vi "UART_SimpleExample.vi"() -> ()   [LabVIEW 2024, in "UART.lvlib"]
doc: "Simple example that shows how to send a command to the DUT and receive the response.\nThe DUT is powered up using a channel from the NI 657x board.\nThe command is sent in the form of Byte Array to be more generic as possible.\nThe response is also received an the form of Byte Array to be more generic as possible"
uses:
  UART.lvlib
panel:
  in  "Input Bytes":u8[](array[numeric])=[1, 3, 12, 0] format="%x"
  out "pass":bool[](array[boolean])=[TRUE]
  out "Reply Bytes":u8[](array[numeric])=[4, 14, 4, 1, 3, 12, 0] format="%x"
  out "error out":errorcluster
  in  "Pattern Label":string="Uart_Main"
  in  "Reply Bytes":i32=7
  in  "EOL Char (Hex)":u8 format="%x"
  in  "Source Buffer":i32=100
  in  "Pin Capture":string="UART_TX_07"
  in  "Pin Source":string="UART_RX_06"
  in  "levels file paths":path[](array[path])=[path "C:/Users/8880_AN/Documents/Customers/STM/657x_UART/DigitalPattern/Levels/LevelsDefault.digilevels"]
  in  "patterns file paths":path[](array[path])=[path "C:/Users/8880_AN/Documents/Customers/STM/657x_UART/DigitalPattern/Pattern/UART_Main.digipat", path "C:/Users/8880_AN/Documents/Customers/STM/657x_UART/DigitalPattern/Pattern/UART_SubCall.digipat"]
  in  "specifications file paths":path[](array[path])=[path "C:/Users/8880_AN/Documents/Customers/STM/657x_UART/DigitalPattern/Specifications/Specifications.specs"]
  in  "pin map file":path=path "C:/Users/8880_AN/Documents/Customers/STM/657x_UART/DigitalPattern/PinMap.pinmap" caption="pin map file path"
  in  "timing file paths":path[](array[path])=[path "C:/Users/8880_AN/Documents/Customers/STM/657x_UART/DigitalPattern/Timing/TimingDefault.digitiming"]
  in  "657x Resource":refnum<k15>="6570"
  # "INPUT PARAMETERS"
  # "RESULTS"
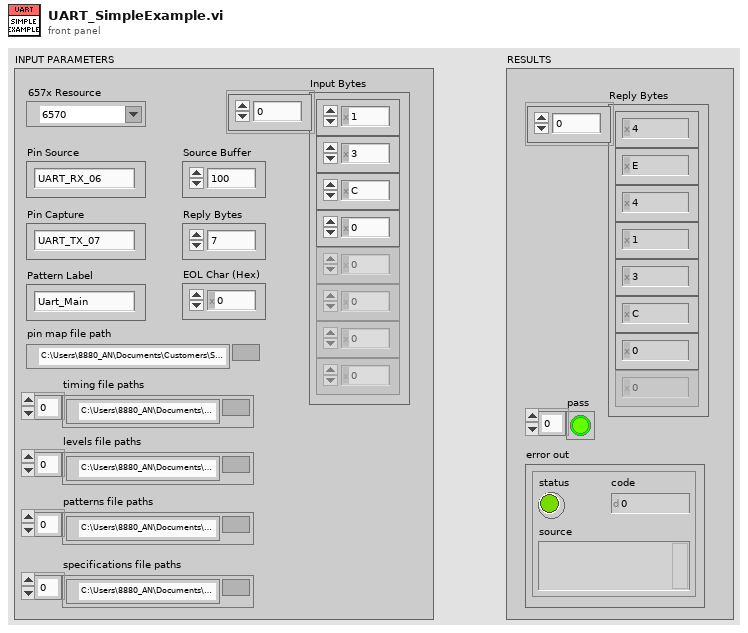
[diagram p1: front panel]
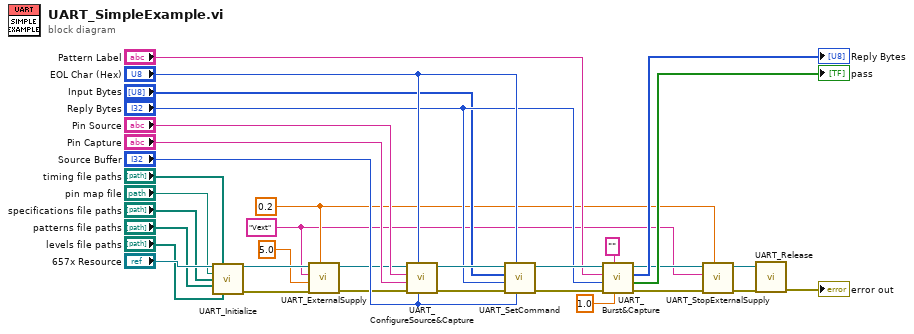
[diagram p0: block diagram]
diagram:
  w2 = 0.2 ("Settling (s)")
  w1 = "Vext" ("Supply Pin")
  n1 = call "UART_Initialize.vi"("resource name"="657x Resource", "timing file paths"="timing file paths", "pin map file"="pin map file", "specifications file paths"="specifications file paths", "patterns file paths"="patterns file paths", "levels file paths"="levels file paths") -> ("instrument handle out"=w10:refnum<k15>, "error out"=w11:errorcluster)  [unwired: 8 in]
  n2 = call "UART_ExternalSupply.vi"("Settling (s)"=w2, "error in (no error)"=w11, "voltage level (V)"=5.0, "Supply Pin"=w1, "IVI Refnum in"=w10) -> ("error out"=w5:errorcluster, "IVI Refnum out"=w4:refnum<k15>)  [unwired: 5 in]
  n3 = call "UART_ConfigureSource&Capture.vi"("Source Buffer"="Source Buffer", "EOL Char (Hex)"="EOL Char (Hex)", "error in (no error)"=w5, "Pin Capture"="Pin Capture", "Pin Source"="Pin Source", "IVI Refnum in"=w4) -> ("error out"=w33:errorcluster, "IVI Refnum out"=w31:refnum<k15>)  [unwired: 4 in]
  n4 = call "UART_SetCommand.vi"("Source Buffer"="Source Buffer", "EOL Char (Hex)"="EOL Char (Hex)", "error in (no error)"=w33, "Reply Bytes"="Reply Bytes", "Command Byte Array"="Input Bytes", "IVI Refnum in"=w31) -> ("error out"=w32:errorcluster, "IVI Refnum out"=w30:refnum<k15>)  [unwired: 4 in]
  n5 = call "UART_Burst&Capture.vi"("timeout (s)"=1.0, "site list"="", "error in (no error)"=w32, "Reply Bytes"="Reply Bytes", "start label"="Pattern Label", "IVI Refnum in"=w30) -> ("error out"=w9:errorcluster, "pass"=→"pass":bool[], "Data Out"=→"Reply Bytes":u8[], "IVI Refnum out"=w8:refnum<k15>)  [unwired: 2 in]
  n6 = call "UART_StopExternalSupply.vi"("Setling (s)"=w2, "error in (no error)"=w9, "pin"=w1, "IVI Refnum in"=w8) -> ("error out"=w6:errorcluster, "IVI Refnum out"=w7:refnum<k15>)  [unwired: 6 in]
  n7 = call "UART_Release.vi"("error in"=w6, "instrument handle"=w7) -> ("error out"=→"error out":errorcluster)  [unwired: 9 in]
